vi "Indicators Temperature Converter.vi"() -> ()   [LabVIEW 2019]
panel:
  in  "Celsius":dbl(slide) scale=0.0..100.0
  out "Kelvin":dbl(slide) scale=273.0..373.0
  out "Fahrenheit":dbl(slide) scale=0.0..212.0
  # "Challenge:\nCreate a temperature converter that converts  a temperature in degrees Celsius to degrees Kelvin and degrees Fahrenheit. Display each temperature on an appropriately scaled thermometer."
  # "Try it: Choose a Celsius temperature and run the program."
  # "You will probably need:\nIndicators and controls, numeric functions"
  # "Open the block diagram to see a possible solution."
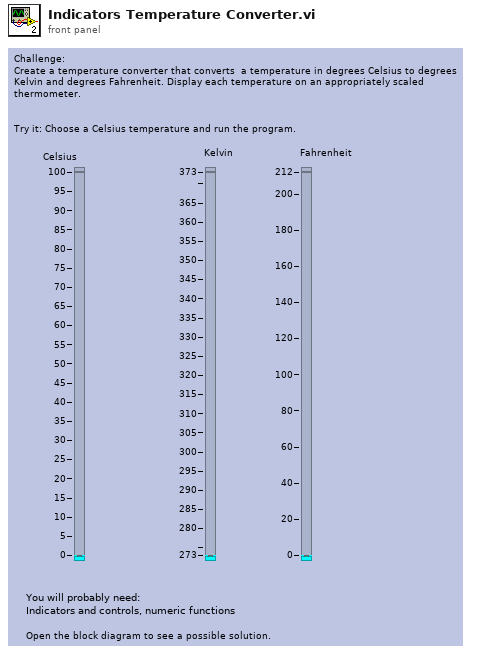
[diagram p1: front panel]
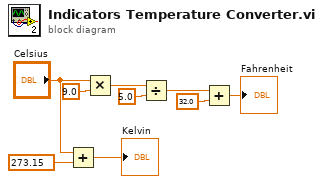
[diagram p0: block diagram]
diagram:
  n1 = Add(x="Celsius", y=273.15) -> (x+y=→"Kelvin":dbl)
  n2 = Multiply(x="Celsius", y=9.0) -> (x*y=w6:dbl)
  n3 = Divide(x=w6, y=5.0) -> (x/y=w5:dbl)
  n4 = Add(x=w5, y=32.0) -> (x+y=→"Fahrenheit":dbl)
